vi "svc_Get Tachometer Channel Info.vi"(0 "Tachometer Channel in":waveform(dbl)) -> (3 "rotation direction":u16(ring) items=["CCW", "CW"], 4 "Tachometer Channel out":waveform(dbl), 6 "Threshold":dbl, 8 "Pulses Per Rev":i32, 12 "Max Order":i32, 13 "Slope":u16(ring) items=["Rising", "Falling"])   [LabVIEW 2017]
doc: "This VI gets tachometer configuration properties from the tachometer waveform attributes."
uses:
  <vilib>/addons/_NISVFA/_Shared subVIs/Controls/SV Channel Properties.ctl
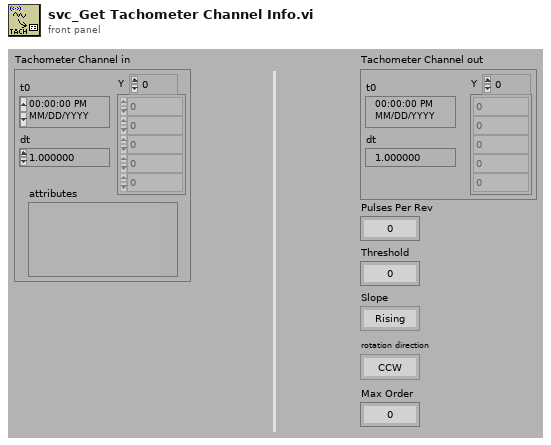
[diagram p1: front panel]
types:
  T1 = typedef "SV Channel Properties.ctl" = u16
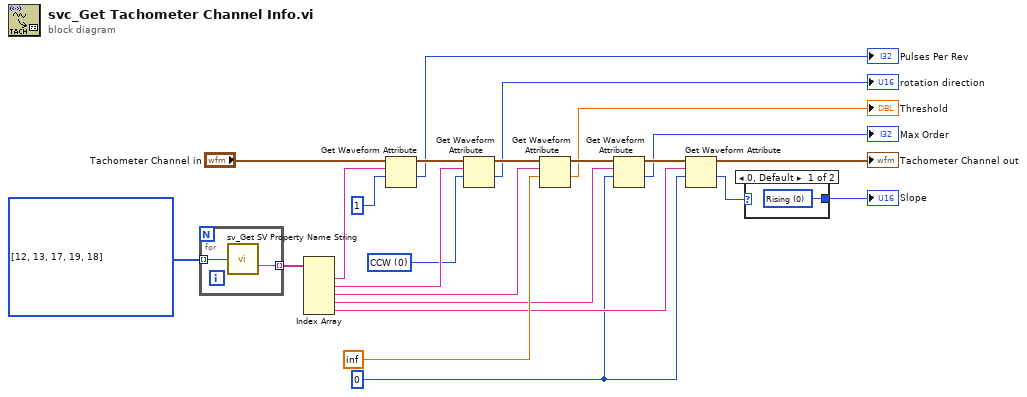
[diagram p0: block diagram]
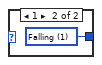
[diagram p2: hidden frame]
diagram:
  w1 = u16 0 items=["CCW", "CW"] ("rotation direction")
  w5 = 0
  w23 = T1[] [12, 13, 17, 19, 18] items=["Engineering units", "Custom unit label", "Weighting filter", "Pregain", "Octave standard", "Octave bandwidth", "Octave low band", "Octave high band", "Spectrum skewed", "Samples / revolution", "Order", "Tachometer", "Pulses Per Revolution", "Rotation Direction", "Probe Angle", "Pair", "Channel Alias", "Tachometer Threshold", "Tachometer Slope", "Max Order", "Sensor Location", "Sensor Orientation"]
  n1 = for {
    tunnel: w23 -> [w25] mode=indexing
    tunnel: [w24] -> w22 mode=indexing
    n2 = call <vilib>:"sv_Get SV Property Name String.vi"("property"=w25) -> ("WDT attribute name"=w24:string)  [unwired: 13 in, 1 out]
  }
  n3 = Index Array(array=w22) -> (element #1=w15:string, element #2=w13:string, element #3=w12:string, element #4=w10:string, element #5=w9:string)  [unwired: 5 in]
  n4 = Get Waveform Attribute(5:1, 6:w15, 7:"Tachometer Channel in") -> (1:→"Pulses Per Rev":i32, 3:w21:waveform(dbl))  [unwired: 1 in, 2 out]
  n5 = Get Waveform Attribute(5:w1, 6:w13, 7:w21) -> (1:→"rotation direction":u16, 3:w20:waveform(dbl))  [unwired: 1 in, 2 out]
  n6 = Get Waveform Attribute(5:inf, 6:w12, 7:w20) -> (1:→"Threshold":dbl, 3:w19:waveform(dbl))  [unwired: 1 in, 2 out]
  n7 = Get Waveform Attribute(5:w5, 6:w10, 7:w19) -> (1:→"Max Order":i32, 3:w18:waveform(dbl))  [unwired: 1 in, 2 out]
  n8 = Get Waveform Attribute(5:w5, 6:w9, 7:w18) -> (1:w4:i32, 3:→"Tachometer Channel out":waveform(dbl))  [unwired: 1 in, 2 out]
  n9 = case shown="0, Default" w4 {
    tunnel: [w26 w27] -> w3
    frame 0, Default {
      w26 = u16 0 items=["Rising", "Falling"] ("slope (Rising)")
    }
    frame 1 {
      w27 = u16 1 items=["Rising", "Falling"] ("slope (Rising)")
    }
  }
  "Slope" <- w3
